vi "Derivative (multiple).vi"(8 "error in (no error)":errorcluster, 10 "Numeric":dbl, 11 "Multiple XY-data in":cluster{"X-array":dbl[], "Y-array":dbl[]}[](array[cluster]) {"Y-array" format="%.2p"; "X-array" format="%.2p"}) -> (0 "error out":errorcluster, 3 "Multiple XY-data out":cluster{"X-array":dbl[], "Y-array":dbl[]}[](array[cluster]) {"Y-array" format="%.2p"; "X-array" format="%.2p"})   [LabVIEW 2016, in "xy_utilities.lvlib"]
uses:
  xy_utilities.lvlib
panel:
  in  "type":enum16{"dy/dx vs x", "dx/dy vs y"}(ring)
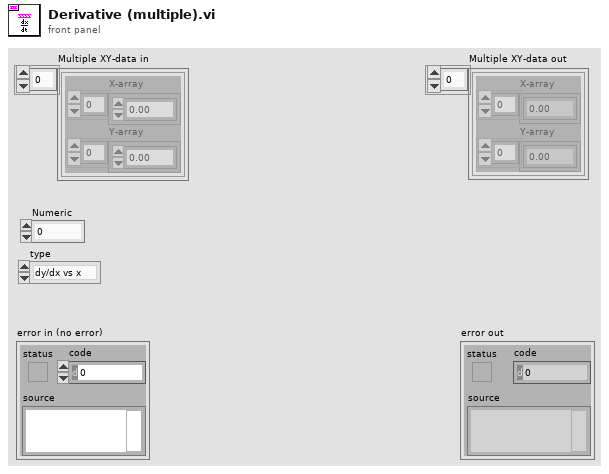
[diagram p1: front panel]
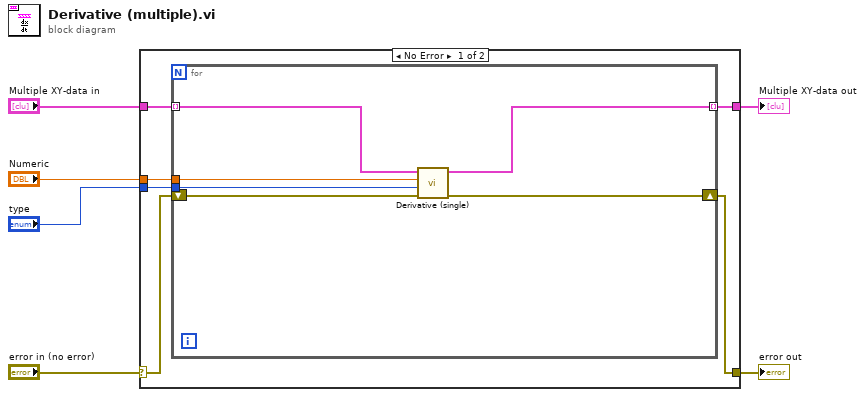
[diagram p0: block diagram]
diagram:
  n1 = case shown="No Error" "error in (no error)" {
    selector: "error in (no error)" -> [w10 w20]
    tunnel: [w9 w20] -> w5
    tunnel: "Multiple XY-data in" -> [w12 w19]
    tunnel: [w11 w19] -> w3
    tunnel: "type" -> [w8 _]
    tunnel: "Numeric" -> [w7 _]
    frame No Error {
      n2 = for {
        tunnel: w12 -> [w16] mode=indexing
        tunnel: [w15] -> w11 mode=indexing
        shift-right: [w17] -> w9
        shift-left: w10 -> [w18]
        tunnel: w8 -> [w14]
        tunnel: w7 -> [w13]
        n3 = call "Derivative (single).vi"("error in (no error)"=w18, "type"=w14, "Numeric"=w13, "XY-data in"=w16) -> ("error out"=w17:errorcluster, "XY-data out"=w15:cluster{"X-array":dbl[], "Y-array":dbl[]})  [unwired: 6 in]
      }
    }
    frame Error {
    }
  }
  "error out" <- w5
  "Multiple XY-data out" <- w3
